vi "LogVersionInfo.vi"(8 "error in (no error)":errorcluster) -> (0 "error out":errorcluster)   [LabVIEW 2018]
uses:
  419b6957-e790-4b1d-9f20-48fbdcfdec14.vi
  089fd608-aedd-428e-844a-b2a123fd7199.vi
  b7ed1d7a-f937-44e9-b280-3097d02dc4bb.vi
  f6a1d7ed-cff8-43dd-8bba-d51f103d5a44.vi
  7a31bf92-c4d5-4832-af94-de0b465b4ea4.vi
  419b6957-e790-4b1d-9f20-48fbdcfdec14.vi/606fffcf-8387-445e-a370-53d8036227eb.vi
  089fd608-aedd-428e-844a-b2a123fd7199.vi/e5faaa12-3fa2-43d7-bd0f-7623f017b58e.vi
  b7ed1d7a-f937-44e9-b280-3097d02dc4bb.vi/426b17ff-e110-42f2-a7ca-9245fec59949.vi
  f6a1d7ed-cff8-43dd-8bba-d51f103d5a44.vi/085044e0-bb6f-4f64-9a53-e08845a08ad5.vi
  7a31bf92-c4d5-4832-af94-de0b465b4ea4.vi/81044657-5038-4ebe-b8d6-95852775ea84.vi
panel:
  out "TargetCPU string":string
  out "Application:Version Number":string
  out "Operating System:Detailed Name":string
  out "Operating System:Build Number":string
  out "Application:Target:CPU":T1(ring)
  out "Application:Directory Path":path
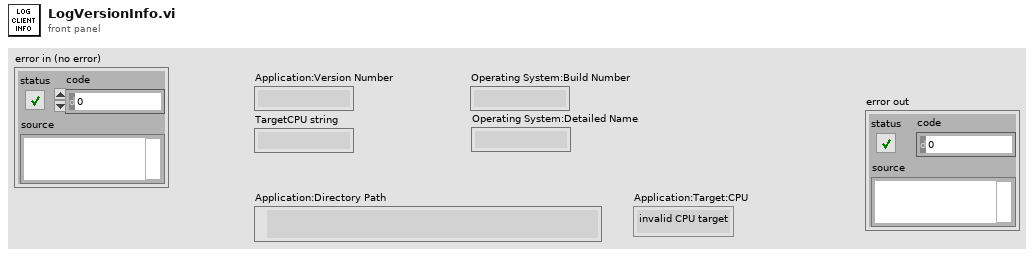
[diagram p1: front panel]
types:
  T1 = enum32{"invalid CPU target", "Motorola 68K", "PowerPC", "Intel x86", "SPARC", "PA-RISC", "MIPS", "Alpha", "ARM", "AMD/Intel x64"}
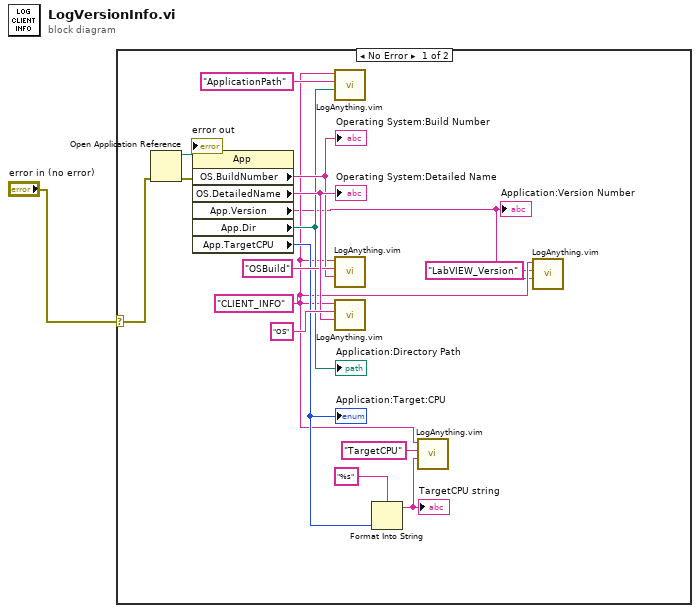
[diagram p0: block diagram]
diagram:
  n1 = case shown="No Error" "error in (no error)" {
    selector: "error in (no error)" -> [w2 _]
    frame No Error {
      w6 = "CLIENT_INFO" ("Category")
      n2 = Open Application Reference(8:w2) -> (0:→"error out":errorcluster, 3:w17:refnum<vi>)  [unwired: 3 in]
      n3 = property class="App"(reference=w17) -> ("OS.BuildNumber"=w11:string, "OS.DetailedName"=w13:string, "App.Version"=w5:string, "App.Dir"=w8:path, "App.TargetCPU"=w7:T1)  [unwired: 1 in, 2 out]
      "Application:Directory Path" <- w8
      "Application:Target:CPU" <- w7
      "Operating System:Build Number" <- w11
      "Operating System:Detailed Name" <- w13
      "Application:Version Number" <- w5
      n4 = call "LogAnything.vim"("Array"=w8, "Var Name"="ApplicationPath", "Category"=w6) -> ()  [unwired: 4 in, 1 out]
      n5 = call "LogAnything.vim"("Array"=w11, "Var Name"="OSBuild", "Category"=w6) -> ()  [unwired: 4 in, 1 out]
      n6 = call "LogAnything.vim"("Array"=w13, "Var Name"="OS", "Category"=w6) -> ()  [unwired: 4 in, 1 out]
      n7 = Format Into String(format string="%s", w7) -> (resulting string=w9:string)  [unwired: 2 in, 1 out]
      "TargetCPU string" <- w9
      n8 = call "LogAnything.vim"("Array"=w9, "Var Name"="TargetCPU", "Category"=w6) -> ()  [unwired: 4 in, 1 out]
      n9 = call "LogAnything.vim"("Array"=w5, "Var Name"="LabVIEW_Version", "Category"=w6) -> ()  [unwired: 4 in, 1 out]
    }
    frame Error {
    }
  }
